vi "U3 Settings Dialog.vi"(8 "error in (no error)":errorcluster, 11 "U3 Module Config in":T2) -> (0 "error out":errorcluster, 1 "Cancelled?":bool=TRUE, 2 "UI Refresh Needed?":bool, 3 "U3 Module Config out":T2)   [LabVIEW 2018, in "U3 Module.lvlib"]
doc: "Dialog for selecting user specified settings."
uses:
  U3 Module.lvlib
  Controls/U3 Module Config Cluster.ctl
  <vilib>/Utility/miscctls.llb/LVPoint32TypeDef.ctl
  Controls/U3 Settings Dialog.ctl
  Shared Variables/Simple Alarm Values Cluster.ctl
  Shared Variables/Dynamic Shared Variables.lvlib
panel:
  in  "Module Name":string
  in  "Settings Dialog":T1 {"AI Channel Number" items=["Default", "AI0", "AI1", "AI2", "AI3", "AI4", "AI5", "AI6", "AI7"]}
  in  "Cancel Button":bool
  in  "OK Button":bool
  # "Non visible portion of dialog (needed for connector pane)."
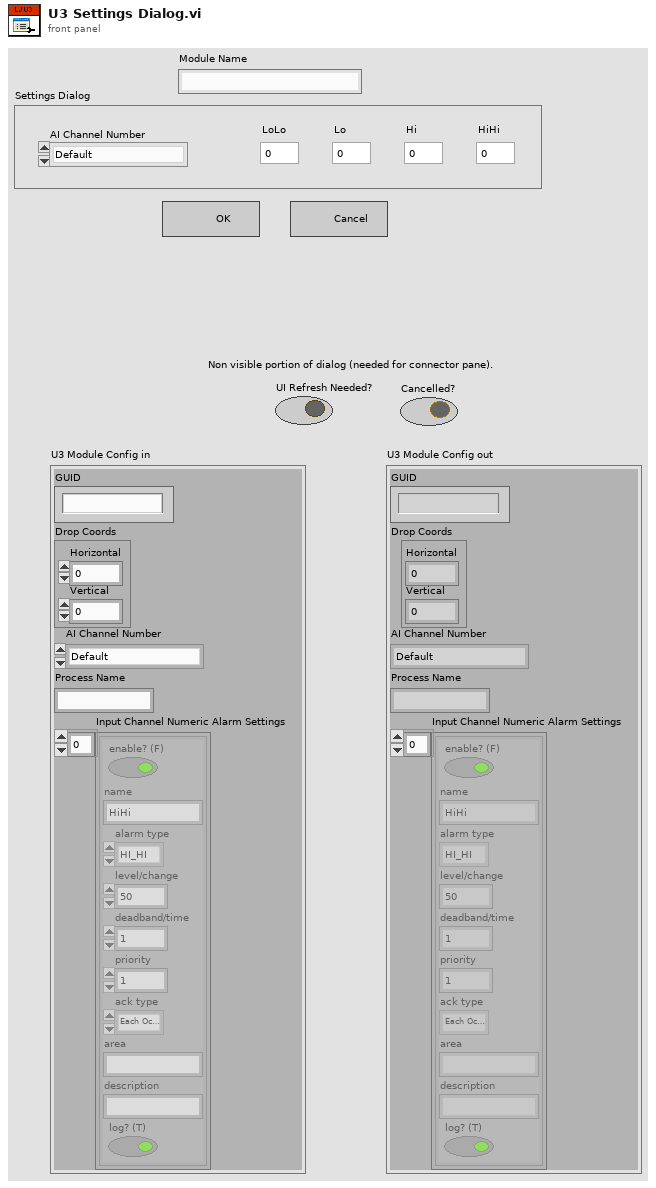
[diagram p1: front panel]
types:
  T1 = typedef "U3 Module.lvlib/U3 Settings Dialog.ctl" = cluster{"AI Channel Number":u16, "LoLo":dbl, "Lo":dbl, "Hi":dbl, "HiHi":dbl}
  T2 = typedef "U3 Module.lvlib/U3 Module Config Cluster.ctl" = cluster{"GUID":string, "Drop Coords":T3, "AI Channel Number":enum16{"Default", "AI0", "AI1", "AI2", "AI3", "AI4", "AI5", "AI6", "AI7"}, "Process Name":string, "Input Channel Numeric Alarm Settings":cluster{"enable? (F)":bool, "name":string, "alarm type":enum16{"HI_HI", "HI", "LO", "LO_LO"}, "level/change":dbl, "deadband/time":dbl, "priority":u32, "ack type":enum16{"Auto", "User", "None", "Each Occurrence"}, "area":string, "description":string, "log? (T)":bool}[]}
  T3 = typedef "LVPoint32TypeDef.ctl" = cluster{"Horizontal":i32, "Vertical":i32}
  T4 = typedef "Dynamic Shared Variables.lvlib/Simple Alarm Values Cluster.ctl" = cluster{"tag name":string, "HiHi":dbl, "Hi":dbl, "Lo":dbl, "LoLo":dbl}
  T5 = enum16{"Default", "AI0", "AI1", "AI2", "AI3", "AI4", "AI5", "AI6", "AI7"}
  T6 = cluster{"enable? (F)":bool, "name":string, "alarm type":enum16{"HI_HI", "HI", "LO", "LO_LO"}, "level/change":dbl, "deadband/time":dbl, "priority":u32, "ack type":enum16{"Auto", "User", "None", "Each Occurrence"}, "area":string, "description":string, "log? (T)":bool}[]
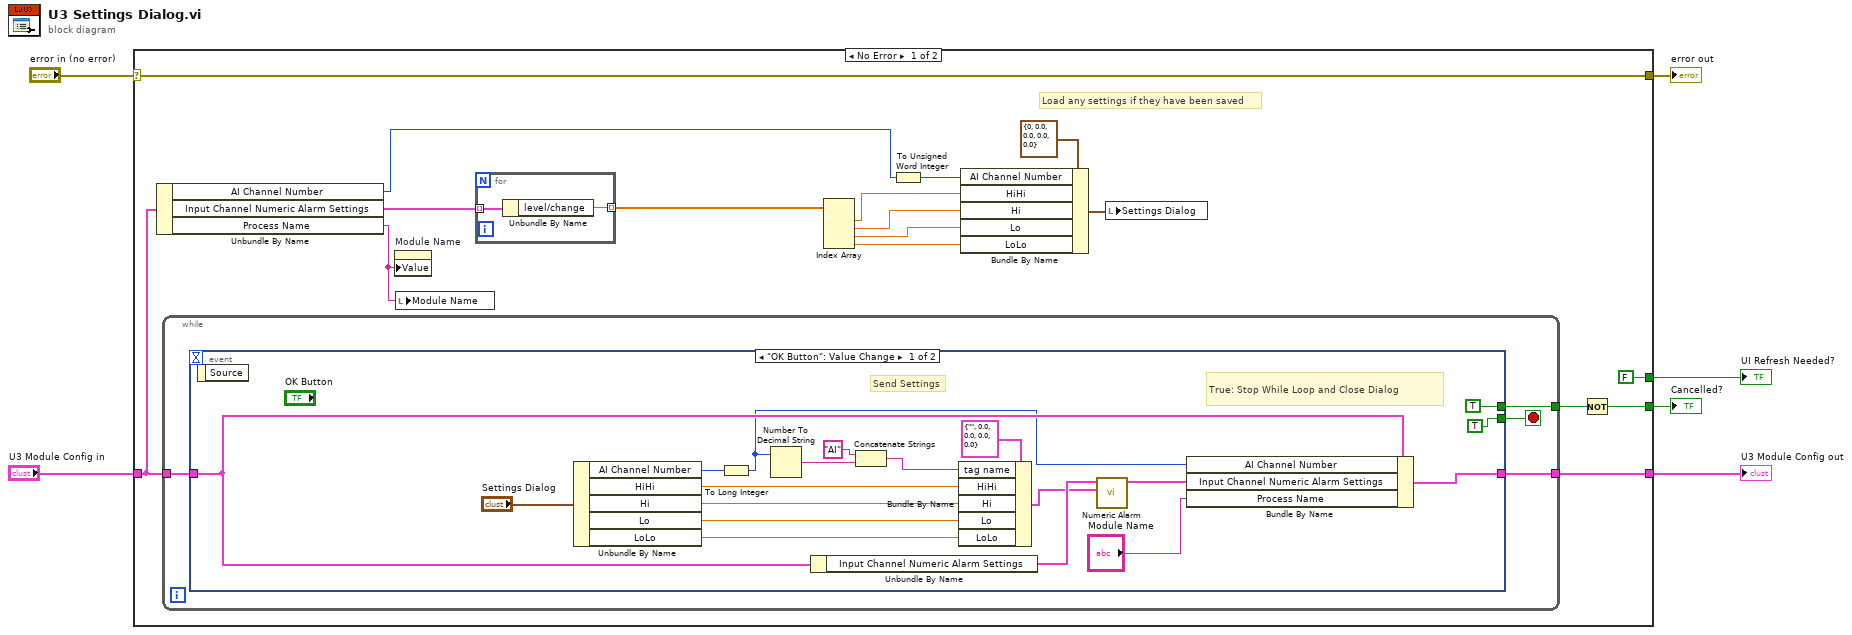
[diagram p0: block diagram]
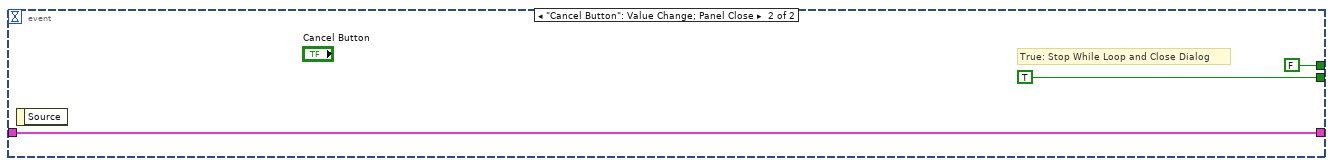
[diagram p2: hidden frame]
diagram:
  n1 = case shown="No Error" "error in (no error)" {
    selector: "error in (no error)" -> [w23 w54]
    tunnel: [w23 w54] -> w6
    tunnel: "U3 Module Config in" -> [w20 w53]
    tunnel: [w21 w53] -> w1
    tunnel: [FALSE ("UI Refresh Needed?") _] -> w4
    tunnel: [w18 TRUE ("UI Refresh Needed?")] -> w3
    frame No Error {
      # "Load any settings if they have been saved"
      n2 = Unbundle By Name(w20) -> ("AI Channel Number"=w8:T5, "Input Channel Numeric Alarm Settings"=w17:T6, "Process Name"=w7:string)
      n3 = while {
        tunnel: [w29] -> w19
        tunnel: [w26] -> w21
        tunnel: w20 -> [w28]
        stop <- w27 stop-if-true
        n4 = event shown="[0] \"OK Button\": Value Change" {
          selector: _ -> [_ _]
          dyn-events: _ -> [_ _]
          timeout: _ -> [_ _]
          tunnel: w28 -> [w43 w51]
          tunnel: [TRUE ("UI Refresh Needed?") FALSE ("UI Refresh Needed?")] -> w29
          tunnel: [TRUE TRUE] -> w27
          tunnel: [w45 w51] -> w26
          event "OK Button": Value Change {
            # "Send Settings"
            # "True: Stop While Loop and Close Dialog"
            n5 = event-data() -> ()  [unwired: 1 in, 1 out]
            n6 = Unbundle By Name("Settings Dialog") -> ("AI Channel Number"=w44:u16, "HiHi"=w40:dbl, "Hi"=w39:dbl, "Lo"=w38:dbl, "LoLo"=w37:dbl)
            n7 = To Long Integer(number=w44) -> (32bit integer=w31:i32)
            n8 = Number To Decimal String(number=w31) -> (decimal integer string=w33:string)  [unwired: 1 in]
            n9 = Unbundle By Name(w43) -> ("Input Channel Numeric Alarm Settings"=w42:T6)
            n10 = Concatenate Strings("AI", w33) -> (w32:string)
            n11 = Bundle By Name(cluster=T4 {"tag name"="", "HiHi"=0.0, "Hi"=0.0, "Lo"=0.0, "LoLo"=0.0} ("Simple Alarm Values"), "tag name"=w32, "HiHi"=w40, "Hi"=w39, "Lo"=w38, "LoLo"=w37) -> (w35:T4)
            n12 = call "Numeric Alarm.vi"("Simple Alarm Values"=w35, "Alarms in"=w42) -> ("Alarms out"=w41:T6)  [unwired: 9 in]
            n13 = Bundle By Name(cluster=w43, "AI Channel Number"=w31, "Input Channel Numeric Alarm Settings"=w41, "Process Name"="Module Name") -> (w45:T2)
          }
          event "Cancel Button": Value Change; Panel Close {
            # "True: Stop While Loop and Close Dialog"
            n14 = event-data() -> ()  [unwired: 1 in, 1 out]
          }
        }
      }
      n15 = property on="Module Name" class="Str"("Value"=w7) -> ()  [unwired: 2 in, 2 out]
      n16 = local write "Module Name"(w7) -> ()
      n17 = for {
        tunnel: w17 -> [w25] mode=indexing
        tunnel: [w24] -> w13 mode=indexing
        n18 = Unbundle By Name(w25) -> ("level/change"=w24:dbl)
      }
      n19 = Index Array(array=w13) -> (element #1=w12:dbl, element #2=w11:dbl, element #3=w10:dbl, element #4=w9:dbl)  [unwired: 4 in]
      n20 = To Unsigned Word Integer(number=w8) -> (unsigned 16bit integer=w15:u16)
      n21 = Bundle By Name(cluster=T1 {"AI Channel Number"=0, "LoLo"=0.0, "Lo"=0.0, "Hi"=0.0, "HiHi"=0.0} ("Settings Dialog"), "AI Channel Number"=w15, "HiHi"=w12, "Hi"=w11, "Lo"=w10, "LoLo"=w9) -> (w14:T1)
      n22 = local write "Settings Dialog"(w14) -> ()
      n23 = Not(x=w19) -> (.not. x?=w18:bool)
    }
    frame Error {
    }
  }
  "UI Refresh Needed?" <- w4
  "error out" <- w6
  "U3 Module Config out" <- w1
  "Cancelled?" <- w3
